vi "Sensor_output.vi"(6 "Sensor Box":string(combo), 7 "Sensors":string, 8 "ED33":string) -> (2 "Sensors_output":string[](array[string]), 3 "ED33_output":string[](array[string]))   [LabVIEW 2013]
panel:
  out "Hall_Z":string
  out "Hall_Y":string
  out "Hall_X":string
  out "KMT39_Cos":string
  out "KMT39_Sin":string
  out "1000_Cos":string
  out "1000_Sin":string
  out "2000_Cos":string
  out "2000_Sin":string
  out "5000_Cos":string
  out "5000_Sin":string
  out "Encoder1":string
  out "Encoder2":string
  out "Timer":string
  out "Version":string
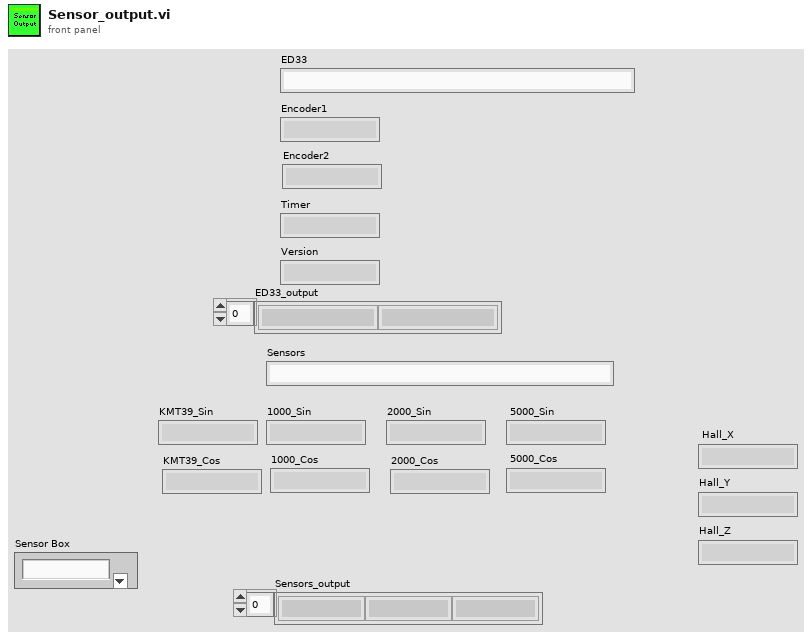
[diagram p1: front panel]
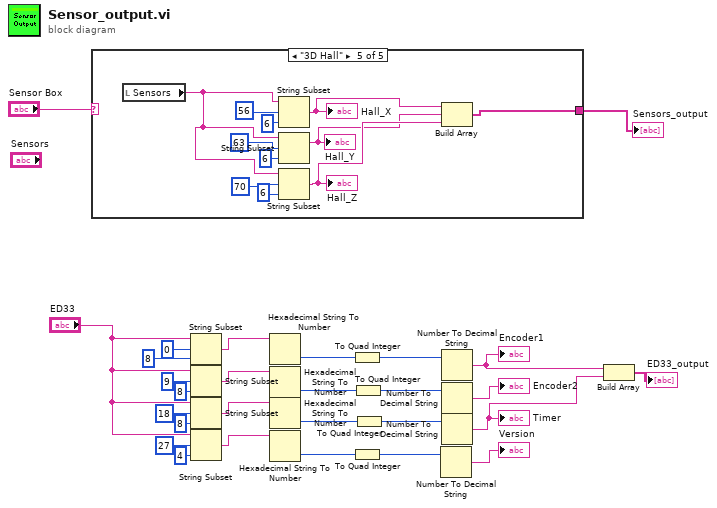
[diagram p0: block diagram]
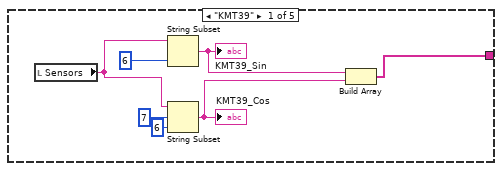
[diagram p2: hidden frame]
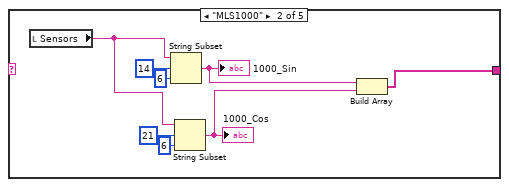
[diagram p3: hidden frame]
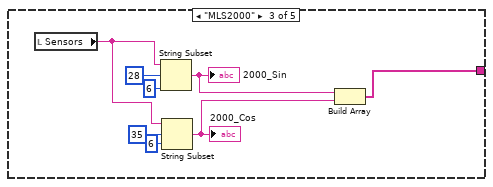
[diagram p4: hidden frame]
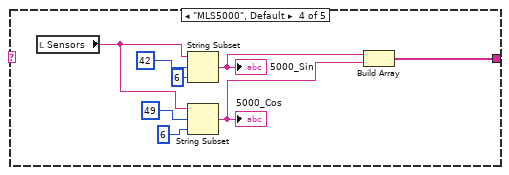
[diagram p5: hidden frame]
diagram:
  n1 = case shown="\"3D Hall\"" "Sensor Box" {
    tunnel: [w29 w37 w44 w53 w60] -> w2
    frame "KMT39" {
      n2 = local read "Sensors"() -> (w32:string)
      n3 = String Subset(string=w32, length (rest)=6 ("Länge (Rest)")) -> (substring=w30:string)  [unwired: 1 in]
      "KMT39_Sin" <- w30
      n4 = String Subset(string=w32, offset (0)=7 ("Offset (0)"), length (rest)=6 ("Länge (Rest)")) -> (substring=w31:string)
      "KMT39_Cos" <- w31
      n5 = Build Array(w30, w31) -> (w29:string[])
    }
    frame "MLS1000" {
      n6 = local read "Sensors"() -> (w36:string)
      n7 = String Subset(string=w36, offset (0)=14 ("Offset (0)"), length (rest)=6 ("Länge (Rest)")) -> (substring=w39:string)
      "1000_Sin" <- w39
      n8 = String Subset(string=w36, offset (0)=21 ("Offset (0)"), length (rest)=6 ("Länge (Rest)")) -> (substring=w38:string)
      "1000_Cos" <- w38
      n9 = Build Array(w39, w38) -> (w37:string[])
    }
    frame "MLS2000" {
      n10 = local read "Sensors"() -> (w45:string)
      n11 = String Subset(string=w45, offset (0)=28 ("Offset (0)"), length (rest)=6 ("Länge (Rest)")) -> (substring=w47:string)
      "2000_Sin" <- w47
      n12 = String Subset(string=w45, offset (0)=35 ("Offset (0)"), length (rest)=6 ("Länge (Rest)")) -> (substring=w46:string)
      "2000_Cos" <- w46
      n13 = Build Array(w47, w46) -> (w44:string[])
    }
    frame "MLS5000", Default {
      n14 = local read "Sensors"() -> (w56:string)
      n15 = String Subset(string=w56, offset (0)=42 ("Offset (0)"), length (rest)=6 ("Länge (Rest)")) -> (substring=w55:string)
      "5000_Sin" <- w55
      n16 = String Subset(string=w56, offset (0)=49 ("Offset (0)"), length (rest)=6 ("Länge (Rest)")) -> (substring=w54:string)
      "5000_Cos" <- w54
      n17 = Build Array(w55, w54) -> (w53:string[])
    }
    frame "3D Hall" {
      n18 = local read "Sensors"() -> (w64:string)
      n19 = String Subset(string=w64, offset (0)=56 ("Offset (0)"), length (rest)=6 ("Länge (Rest)")) -> (substring=w61:string)
      "Hall_X" <- w61
      n20 = String Subset(string=w64, offset (0)=63 ("Offset (0)"), length (rest)=6 ("Länge (Rest)")) -> (substring=w62:string)
      "Hall_Y" <- w62
      n21 = String Subset(string=w64, offset (0)=70 ("Offset (0)"), length (rest)=6 ("Länge (Rest)")) -> (substring=w63:string)
      "Hall_Z" <- w63
      n22 = Build Array(w61, w62, w63) -> (w60:string[])
    }
  }
  "Sensors_output" <- w2
  n23 = String Subset(string="ED33", offset (0)=0 ("Offset (0)"), length (rest)=8 ("Länge (Rest)")) -> (substring=w25:string)
  n24 = String Subset(string="ED33", offset (0)=9 ("Offset (0)"), length (rest)=8 ("Länge (Rest)")) -> (substring=w26:string)
  n25 = String Subset(string="ED33", offset (0)=18 ("Offset (0)"), length (rest)=8 ("Länge (Rest)")) -> (substring=w27:string)
  n26 = String Subset(string="ED33", offset (0)=27 ("Offset (0)"), length (rest)=4 ("Länge (Rest)")) -> (substring=w28:string)
  n27 = Hexadecimal String To Number(string=w25) -> (number=w7:u32)  [unwired: 2 in, 1 out]
  n28 = Hexadecimal String To Number(string=w26) -> (number=w8:u32)  [unwired: 2 in, 1 out]
  n29 = Hexadecimal String To Number(string=w27) -> (number=w9:u32)  [unwired: 2 in, 1 out]
  n30 = Hexadecimal String To Number(string=w28) -> (number=w11:u32)  [unwired: 2 in, 1 out]
  n31 = To Quad Integer(1:w7) -> (0:w6:i64)
  n32 = To Quad Integer(1:w11) -> (0:w10:i64)
  n33 = To Quad Integer(1:w8) -> (0:w5:i64)
  n34 = To Quad Integer(1:w9) -> (0:w4:i64)
  n35 = Number To Decimal String(number=w10) -> (decimal integer string=→"Version":string)  [unwired: 1 in]
  n36 = Number To Decimal String(number=w6) -> (decimal integer string=w16:string)  [unwired: 1 in]
  "Encoder1" <- w16
  n37 = Number To Decimal String(number=w5) -> (decimal integer string=→"Encoder2":string)  [unwired: 1 in]
  n38 = Number To Decimal String(number=w4) -> (decimal integer string=w1:string)  [unwired: 1 in]
  "Timer" <- w1
  n39 = Build Array(w16, w1) -> (→"ED33_output":string[])
